vi "ReadTestData.vi"(10 "settings_um":i32[](array[numeric]), 11 "settings_aod":i32[](array[numeric])) -> (1 "coordinates":dbl[][](array[numeric]), 2 "linearvolume":dbl[][](array[numeric]), 3 "testdata":dbl[][](array[numeric]))   [LabVIEW 2014]
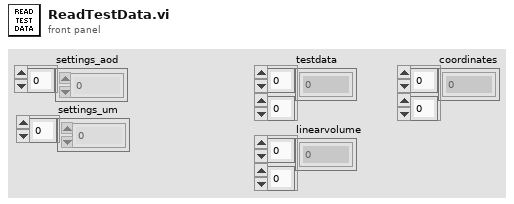
[diagram p1: front panel]
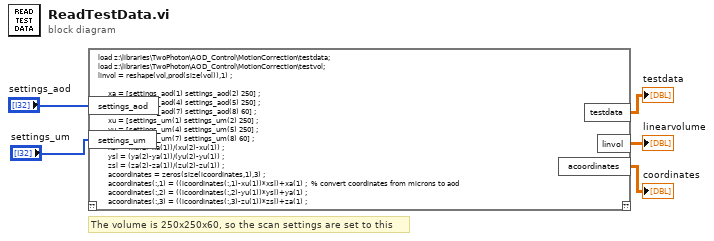
[diagram p0: block diagram]
diagram:
  # "The volume is 250x250x60, so the scan settings are set to this"
  n1 = script code="load z:\\libraries\\TwoPhoton\\AOD_Control\\MotionCorrection\\testdata;\nload z:\\libraries\\TwoPhoton\\AOD_Control\\MotionCorrection\\testvol;\nlinvol = reshape(vol,prod(size(vol)),1) ;\n\n     xa = [settings_aod(1) settings_aod(2) 250] ;\n     ya = [settings_aod(4) settings_aod(5) 250] ;\n     za = [settings_aod(7) settings_aod(8) 60] ;\n     xu = [settings_um(1) settings_um(2) 250] ;\n     yu = [settings_um(4) settings_um(5) 250] ;\n     zu = [settings_um(7) settings_um(8) 60] ;\n     xsl = (xa(2)-xa(1))/(xu(2)-xu(1)) ;\n     ysl = (ya(2)-ya(1))/(yu(2)-yu(1)) ;\n     zsl = (za(2)-za(1))/(zu(2)-zu(1)) ;\n     acoordinates = zeros(size(icoordinates,1),3) ;\n     acoordinates(:,1) = ((icoordinates(:,1)-xu(1))*xsl)+xa(1) ;  % convert coordinates from microns to aod\n     acoordinates(:,2) = ((icoordinates(:,2)-yu(1))*ysl)+ya(1) ;\n     acoordinates(:,3) = ((icoordinates(:,3)-zu(1))*zsl)+za(1) ;"("settings_aod"="settings_aod", "settings_um"="settings_um") -> ("testdata"=→"testdata":dbl[][], "linvol"=→"linearvolume":dbl[][], "acoordinates"=→"coordinates":dbl[][])  [unwired: 1 in, 1 out]
